vi "write_attributes.vi"(8 "error in (no error)":errorcluster, 10 "attributes":T1, 11 "ExtraTreeClassifier in":refnum<class "ExtraTreeClassifier.lvclass">) -> (0 "error out":errorcluster, 3 "ExtraTreeClassifier out":refnum<class "ExtraTreeClassifier.lvclass">)   [LabVIEW 2020, in "ExtraTreeClassifier.lvclass"]
uses:
  ExtraTreeClassifier.lvclass
  Controls/extra_tree_classifier_attributes.ctl
  ExtraTreeClassifier.lvclass/ExtraTreeClassifier.ctl
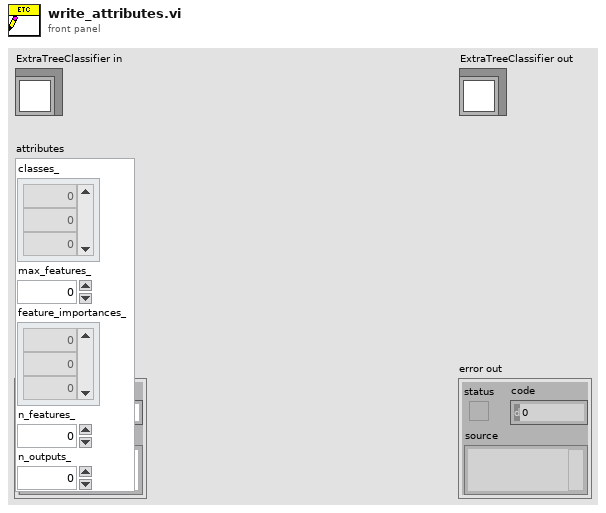
[diagram p1: front panel]
types:
  T1 = typedef "extra_tree_classifier_attributes.ctl" = cluster{"classes_":dbl[][], "max_features_":dbl, "feature_importances_":dbl[], "n_features_":dbl, "n_outputs_":dbl}
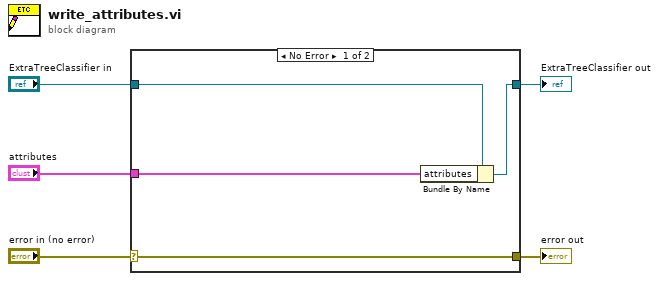
[diagram p0: block diagram]
diagram:
  n1 = case shown="No Error" "error in (no error)" {
    selector: "error in (no error)" -> [w9 w10]
    tunnel: [w9 w10] -> w4
    tunnel: [w7 w11] -> w2
    tunnel: "ExtraTreeClassifier in" -> [w8 w11]
    tunnel: "attributes" -> [w6 _]
    frame No Error {
      n2 = Bundle By Name(cluster=w8, "attributes"=w6) -> (w7:refnum<class "ExtraTreeClassifier.lvclass">)
    }
    frame Error {
    }
  }
  "error out" <- w4
  "ExtraTreeClassifier out" <- w2
